vi "vel.vi"() -> ()   [LabVIEW 2019]
panel:
  in  "Boolean":bool
  out "Enc":dbl[](array[numeric])
  out "power":dbl[](array[numeric])
  out "®t­È":dbl[](array[numeric])
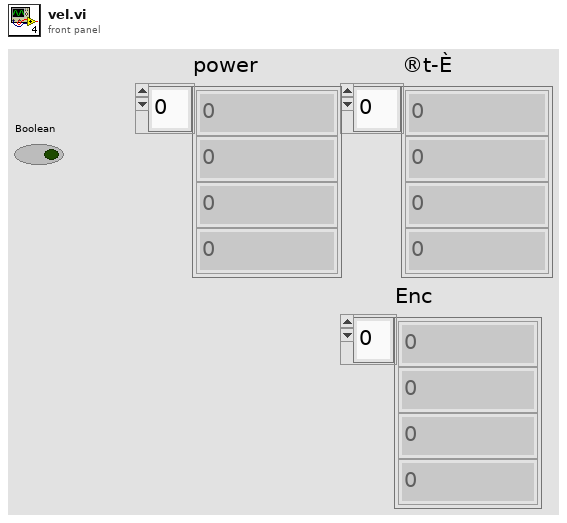
[diagram p1: front panel]
types:
  T1 = cluster{"proportional gain (Kc)":dbl, "integral time (Ti, min)":dbl, "derivative time (Td, min)":dbl}
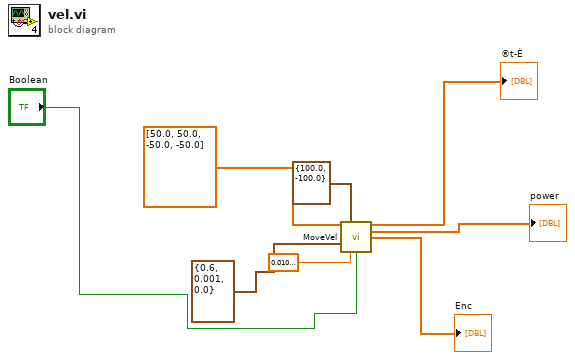
[diagram p0: block diagram]
diagram:
  n1 = call "MoveVel.vi"("OBJ"=dbl[] [50.0, 50.0, -50.0, -50.0], "output range"=cluster{"output high":dbl, "output low":dbl} {"output high"=100.0, "output low"=-100.0}, "PID gains"=T1 {"proportional gain (Kc)"=0.6, "integral time (Ti, min)"=0.001, "derivative time (Td, min)"=0.0}, "dt (s)"=0.010000000000000002, "STOP"="Boolean") -> ("®t­È"=→"®t­È":dbl[], "power"=→"power":dbl[], "Enc"=→"Enc":dbl[])  [unwired: 7 in, 1 out]
